vi "Read Configuration Parameters.vi"(8 "error in (no error)":errorcluster, 10 "refnum":T1, 11 "Step Configuration in":refnum<class "Step Configuration.lvclass">) -> (0 "error out":errorcluster, 2 "refnum out":T1, 3 "Step Configuration out":refnum<class "Step Configuration.lvclass">)   [LabVIEW 2017, in "Measurement Actor.lvlib" / "Step Configuration.lvclass"]
uses:
  Step Configuration.lvclass
  <vilib>/Utility/config.llb/Config Data RefNum.ctl
  Step Configuration.lvclass/Step Configuration.ctl
  <userlib>/Configuration Dialog Actor/Configuration.lvclass
  <vilib>/Utility/config.llb/NI_LVConfig.lvlib
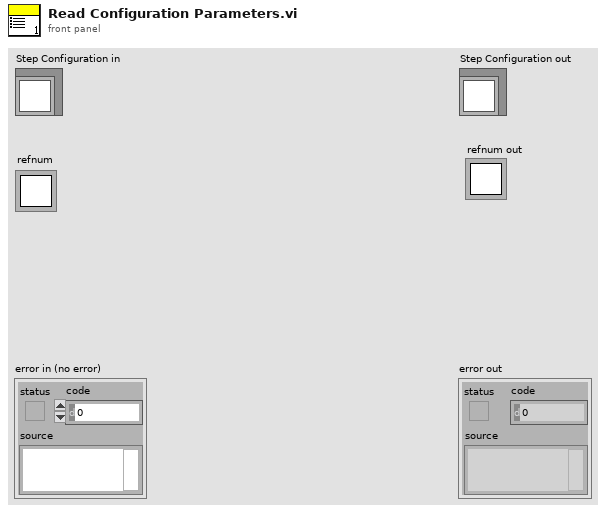
[diagram p1: front panel]
types:
  T1 = typedef "NI_LVConfig.lvlib/Config Data RefNum.ctl" = refnum<k1>
  T2 = cluster{"Run indefinitely":bool, "Iterations":i32}
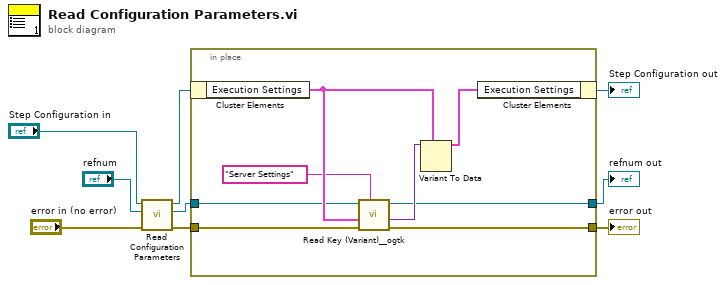
[diagram p0: block diagram]
diagram:
  n1 = call-parent "Read Configuration Parameters.vi"("error in (no error)"="error in (no error)", "refnum"="refnum", "Configuration in"="Step Configuration in") -> ("error out"=w5:errorcluster, "refnum out"=w6:T1, "Configuration out"=w4:refnum<class "Step Configuration.lvclass">)  [unwired: 6 in]
  n2 = in-place {
    in-place-border: w6 -> [w14]
    in-place-border: [w13] -> w2
    in-place-border: w5 -> [w12]
    in-place-border: [w11] -> w1
    n3 = in-place-cluster #1(w4) -> ("Execution Settings"=w17:T2)
    n4 = call <userlib>:"Read Key (Variant)__ogtk.vi"("section"="Server Settings", "error in (no error)"=w12, "type"=w17, "refnum"=w14) -> ("error out"=w11:errorcluster, "key-value"=w16:variant, "refnum out"=w13:T1)  [unwired: 4 in, 1 out]
    n5 = Variant To Data(type=w17, Variant=w16) -> (data=w15:T2)  [unwired: 1 in, 1 out]
    n6 = in-place-cluster #1("Execution Settings"=w15) -> (→"Step Configuration out":refnum<class "Step Configuration.lvclass">)
  }
  "error out" <- w1
  "refnum out" <- w2
